vi "Function A.vi"() -> (2 "String":string)   [LabVIEW 2020, in "Library A.lvlib"]
uses:
  Library A.lvlib
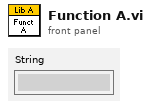
[diagram p1: front panel]
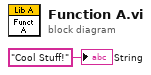
[diagram p0: block diagram]
diagram:
  "String" <- "Cool Stuff!" ("String")
